vi "Express XY图（李萨如图形）.vi"() -> ()   [LabVIEW 2017]
uses:
  <vilib>/measure/NI_MABase.lvlib
panel:
  in  "phase1":dbl
  in  "phase":dbl
  in  "频率 1":dbl
  in  "频率":dbl
  out "XY Graph":cluster{"Y":dbl[], "Y":dbl[]}[](graph) caption="XY图"
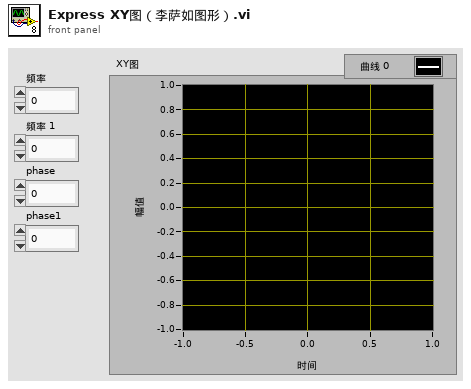
[diagram p1: front panel]
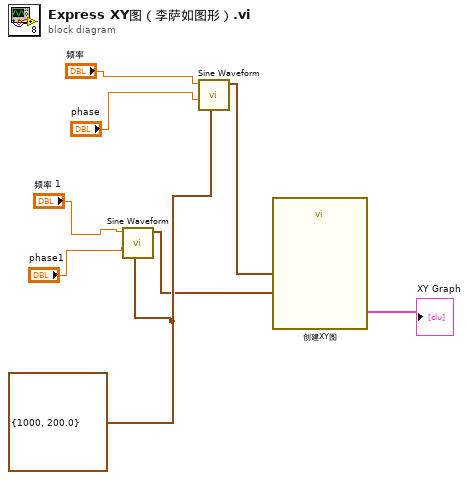
[diagram p0: block diagram]
diagram:
  w3 = cluster{i32, dbl} {1000, 200.0}
  n1 = call <vilib>:"Sine Waveform.vi"("sampling info"=w3, "phase"="phase1", "frequency"="频率 1") -> ("signal out"=w1:waveform(dbl))  [unwired: 7 in, 1 out]
  n2 = call <vilib>:"Sine Waveform.vi"("sampling info"=w3, "phase"="phase", "frequency"="频率") -> ("signal out"=w2:waveform(dbl))  [unwired: 7 in, 1 out]
  n3 = call "创建XY图"("Y Input"=w1, "X Input"=w2) -> ("XY Graph"=→"XY Graph":cluster{"X":dbl[], "Y":dbl[]}[])  [unwired: 8 in, 1 out]
